vi "gwyscan create path space filling progressive.vi"(0 "xypos":dbl[](array[numeric]), 1 "xreal":dbl, 2 "xoffset":dbl, 5 "order":i32, 7 "coarse_order":i32, 9 "skip_order":i32, 11 "error in (no error)":errorcluster, 12 "yreal":dbl, 13 "yoffset":dbl) -> (4 "xypos out":dbl[](array[numeric]), 6 "function return":i32, 15 "error out":errorcluster)   [LabVIEW 2016, in "libgwyscan.lvlib"]
doc: "GWYSCANDLL_API int gwyscan_create_path_space_filling_progressive(double *xypos, int order, int coarse_order, int skip_order, double xreal, double yreal, double xoffset, double yoffset);"
uses:
  libgwyscan.lvlib
  libgwyscan.dll
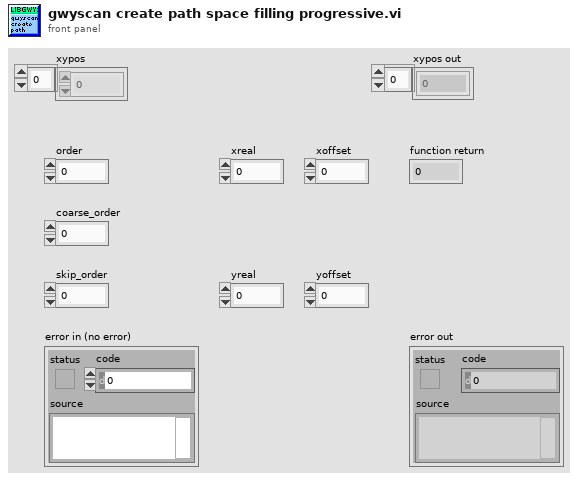
[diagram p1: front panel]
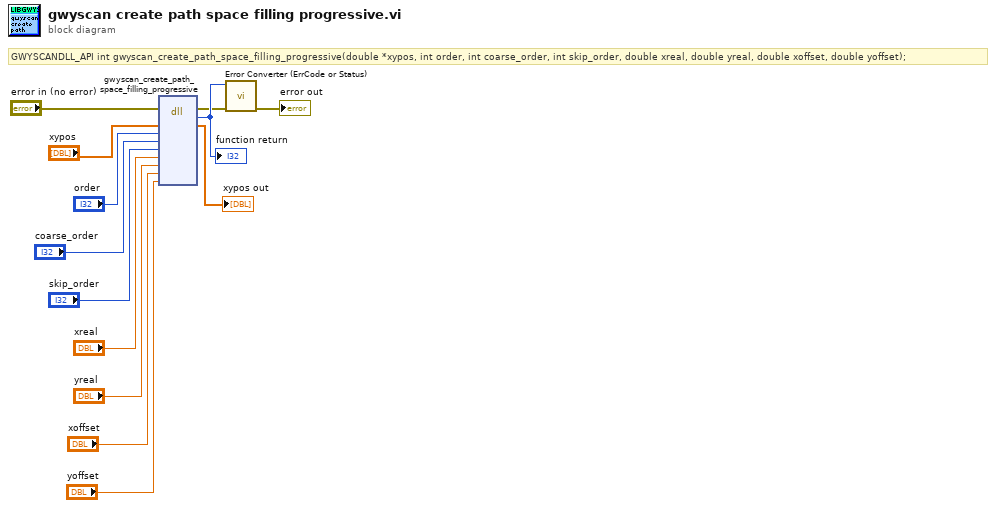
[diagram p0: block diagram]
diagram:
  # "GWYSCANDLL_API int gwyscan_create_path_space_filling_progressive(double *xypos, int order, int coarse_order, int skip_order, double xreal, double yreal, double xoffset, double yoffset);"
  n1 = dll-call lib="PTH2abs CUsersCharlÃ¨ne BrillardDesktoplbni-lbniAFMController-BetaVersionv2.0.16-20190611 libgwyscan-1.2-labview2015-win32libgwyscan.*" fn="gwyscan_create_path_space_filling_progressive"(error in="error in (no error)", "xypos"="xypos", "order"="order", "coarse_order"="coarse_order", "skip_order"="skip_order", "xreal"="xreal", "yreal"="yreal", "xoffset"="xoffset", "yoffset"="yoffset") -> (error out=w3:errorcluster, "return type"=w13:i32, "xypos"=→"xypos out":dbl[])  [unwired: 9 in, 1 out]
  "function return" <- w13
  n2 = call "Error Converter (ErrCode or Status).vi"("error in (no error)"=w3, "error code"=w13) -> ("error out"=→"error out":errorcluster)  [unwired: 9 in]
